vi "_시리얼_Mark10-데이터 수신 (스탠드 상태).vi"(5 "시리얼 포트":refnum<visa-resource-name>="COM5") -> (1 "모터 정지 상태":bool, 2 "시리얼 포트 out":refnum<visa-resource-name>="COM5")   [LabVIEW 2015]
panel:
  out "Process Time(ms)":u32
  out "버퍼 읽기":string
  # "MARK10 게이지 데이터 수신"
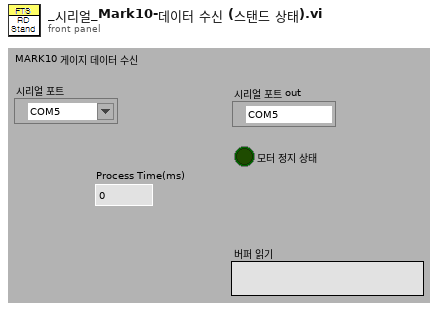
[diagram p1: front panel]
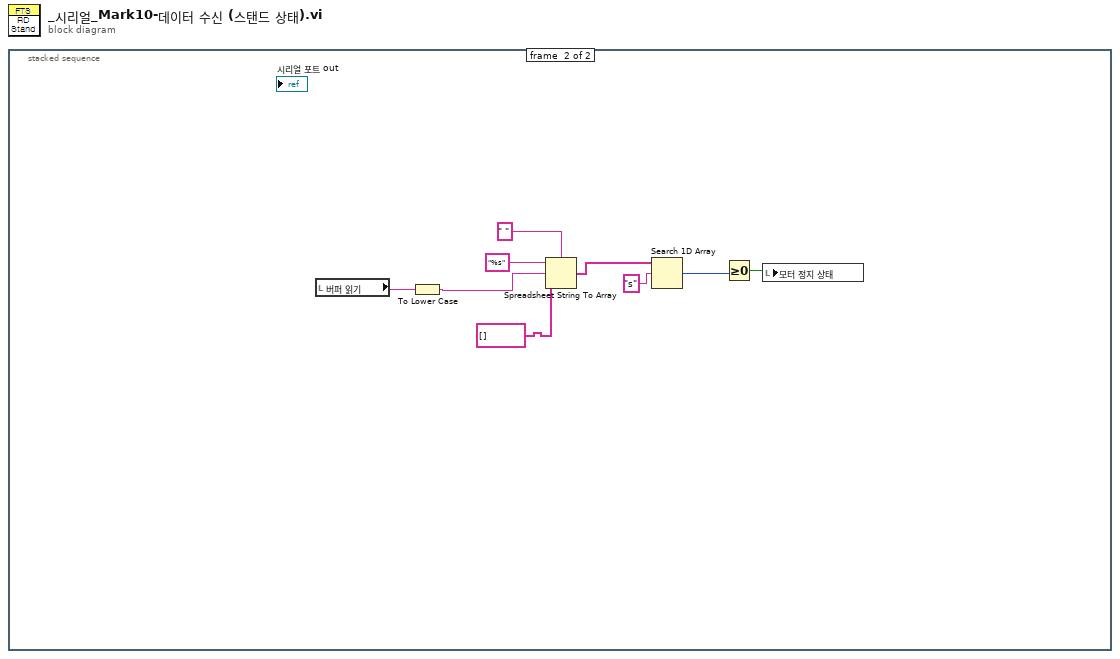
[diagram p0: block diagram]
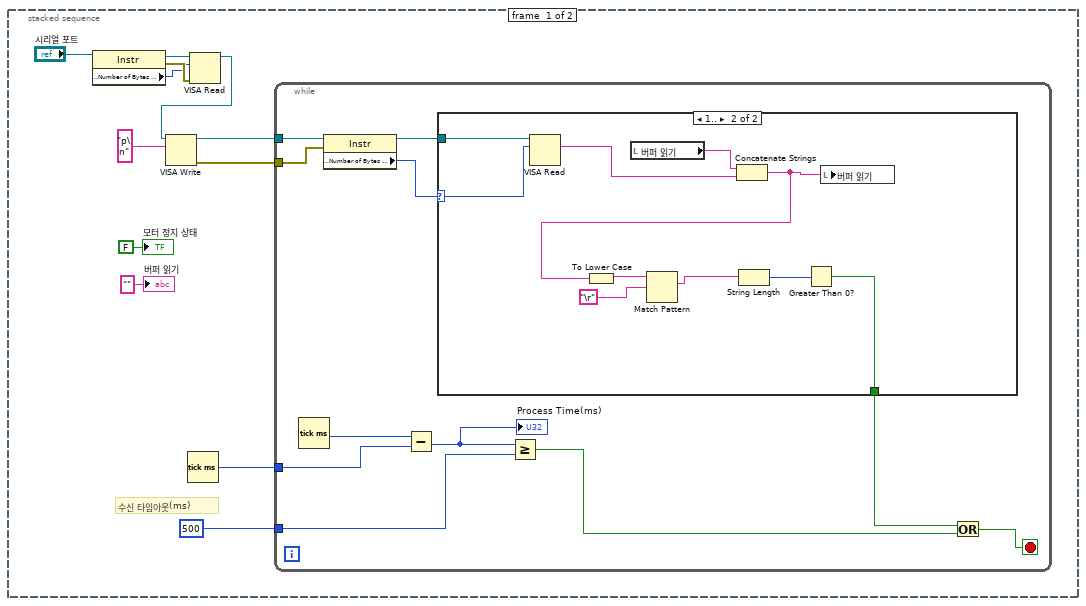
[diagram p2: hidden frame]
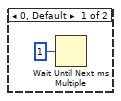
[diagram p3: hidden frame]
diagram:
  n1 = stacked-sequence {
    frame #0 {
      # "수신 타임아웃(ms)"
      n2 = property class="Instr"(reference="시리얼 포트") -> (reference out=w6:refnum<visa-resource-name>, error out=w4:errorcluster, "Serial Settings:Number of Bytes at Serial Port"=w1:u32)  [unwired: 1 in]
      n3 = Tick Count (ms)() -> (millisecond timer value=w8:u32)
      n4 = VISA Read(VISA resource name=w6, byte count=w1, error in (no error)=w4) -> (VISA resource name out=w3:refnum<visa-resource-name>)  [unwired: 3 out]
      n5 = VISA Write(VISA resource name=w3, write buffer="p\n") -> (VISA resource name out=w10:refnum<visa-resource-name>, error out=w9:errorcluster)  [unwired: 1 in, 1 out]
      n6 = while {
        tunnel: w10 -> [w22]
        tunnel: w9 -> [w21]
        tunnel: w8 -> [w18]
        tunnel: 500 -> [w16]
        stop <- w14 stop-if-true
        n7 = Tick Count (ms)() -> (millisecond timer value=w19:u32)
        n8 = property class="Instr"(reference=w22, error in=w21) -> (reference out=w23:refnum<visa-resource-name>, "Serial Settings:Number of Bytes at Serial Port"=w20:u32)  [unwired: 1 out]
        n9 = Subtract(x=w19, y=w18) -> (x-y=w17:u32)
        "Process Time(ms)" <- w17
        n10 = case shown="1.." w20 {
          selector: w20 -> [_ w27]
          tunnel: w23 -> [_ w34]
          tunnel: [_ w28] -> w13
          frame 0, Default {
            n11 = Wait Until Next ms Multiple(millisecond multiple=u32 1 ("ms 배수")) -> ()  [unwired: 1 out]
          }
          frame 1.. {
            n12 = VISA Read(VISA resource name=w34, byte count=w27) -> (read buffer=w32:string)  [unwired: 1 in, 3 out]
            n13 = local read "버퍼 읽기"() -> (w33:string)
            n14 = Concatenate Strings(w33, w32) -> (w31:string)
            n15 = To Lower Case(string=w31) -> (all lower case string=w30:string)
            n16 = Match Pattern(string=w30, regular expression="\r") -> (match substring=w26:string)  [unwired: 1 in, 3 out]
            n17 = String Length(string=w26) -> (length=w29:i32)
            n18 = Greater Than 0?(x=w29) -> (x > 0?=w28:bool)
            n19 = local write "버퍼 읽기"(w31) -> ()
          }
        }
        n20 = Greater Or Equal?(x=w17, y=w16) -> (x >= y?=w15:bool)
        n21 = Or(x=w13, y=w15) -> (x .or. y?=w14:bool)
      }
      "모터 정지 상태" <- FALSE ("수신 정상")
      "버퍼 읽기" <- "" ("버퍼 읽기")
    }
    frame #1 {
      n22 = local read "버퍼 읽기"() -> (w43:string)
      n23 = To Lower Case(string=w43) -> (all lower case string=w40:string)
      n24 = Spreadsheet String To Array(delimiter (Tab)=" " ("구분 문자(탭)"), format string="%s" ("포맷 문자열"), spreadsheet string=w40, array type (2D Dbl)=string[] [] ("배열 타입(2D Dbl)")) -> (array=w38:string[])
      n25 = Search 1D Array(1D array=w38, element="s" ("원소")) -> (index of element=w35:i32)  [unwired: 1 in]
      n26 = Greater Or Equal To 0?(x=w35) -> (x >= 0?=w36:bool)
      n27 = local write "모터 정지 상태"(w36) -> ()
    }
  }
